vi "TETRIX Servo Move_HT_myRIO.vi"(0 "Servo Position (0 - 255)":u8(slide)=128 step=1 scale=0.0..255.0, 1 "Controller Daisy Chain Position (1 - 4)":u8=1, 3 "Enable Sync: Fast | Medium | Slow | None":string(combo)="None", 4 "Select Servo":string(combo)="Servo 1", 5 "error in (no error)":errorcluster) -> (2 "error out":errorcluster)   [LabVIEW 2014]
uses:
  <vilib>/myRIO/Instrument Drivers/Onboard IO/I2C/vis/Configure.vi
  <vilib>/myRIO/Instrument Drivers/Onboard IO/I2C/vis/Write.vi
  <vilib>/myRIO/Instrument Drivers/Onboard IO/I2C/vis/Smart Open.vi
  <vilib>/Utility/error.llb/Error Cluster From Error Code.vi
  <vilib>/myRIO/Common/Instrument Driver Framework/myRIO v1.0/I2C/vis/myRIO v1.0 Configure I2C.vi
  <vilib>/myRIO/Common/Instrument Driver Framework/myRIO v1.0/I2C/vis/myRIO v1.0 Write I2C.vi
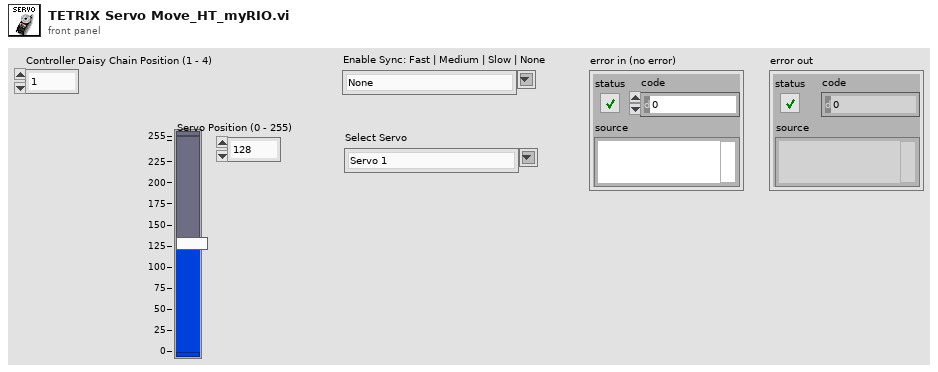
[diagram p1: front panel]
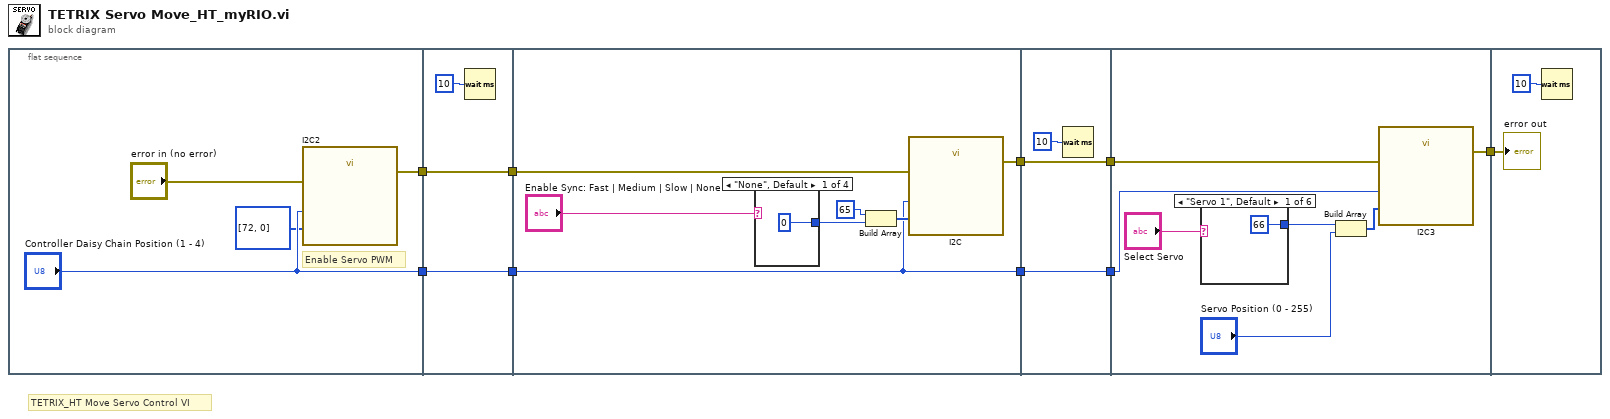
[diagram p0: block diagram]
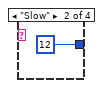
[diagram p2: hidden frame]
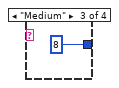
[diagram p3: hidden frame]
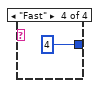
[diagram p4: hidden frame]
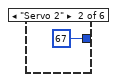
[diagram p5: hidden frame]
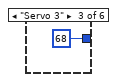
[diagram p6: hidden frame]
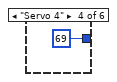
[diagram p7: hidden frame]
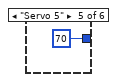
[diagram p8: hidden frame]
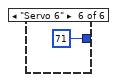
[diagram p9: hidden frame]
diagram:
  # "TETRIX_HT Move Servo Control VI"
  n1 = flat-sequence {
    tunnel: ["Controller Daisy Chain Position (1 - 4)"] -> w9
    tunnel: [w11] -> w7
    tunnel: w9 -> [w16]
    tunnel: [w16] -> w8
    tunnel: w7 -> [w15]
    tunnel: [w15] -> w6
    tunnel: [w19] -> w5
    tunnel: w8 -> [w17]
    tunnel: w6 -> [w18]
    tunnel: [w17] -> w3
    tunnel: w5 -> [w30]
    tunnel: [w30] -> w4
    tunnel: w3 -> [w29]
    tunnel: [w29] -> w2
    tunnel: w4 -> [w32]
    tunnel: w2 -> [w33]
    tunnel: [w31] -> w1
    tunnel: w1 -> [w44]
    frame #0 {
      # "Enable Servo PWM"
      n2 = call "I2C2"("Slave Address (7-bit)"="Controller Daisy Chain Position (1 - 4)", "Bytes to Write"=u8[] [72, 0], "error in (no error)"="error in (no error)") -> ("error out"=w11:errorcluster)  [unwired: 24 in]
    }
    frame #1 {
      n3 = Wait (ms)(milliseconds to wait=u32 10) -> ()  [unwired: 1 out]
    }
    frame #2 {
      n4 = case shown="\"None\", Default" "Enable Sync: Fast | Medium | Slow | None" {
        tunnel: [u8 0 u8 12 u8 8 u8 4] -> w21
        frame "None", Default {
        }
        frame "Slow" {
        }
        frame "Medium" {
        }
        frame "Fast" {
        }
      }
      n5 = Build Array(u8 65 ("element"), w21) -> (w22:u8[])
      n6 = call "I2C"("Slave Address (7-bit)"=w17, "Bytes to Write"=w22, "error in (no error)"=w18) -> ("error out"=w19:errorcluster)  [unwired: 24 in]
    }
    frame #3 {
      n7 = Wait (ms)(milliseconds to wait=u32 10) -> ()  [unwired: 1 out]
    }
    frame #4 {
      n8 = case shown="\"Servo 1\", Default" "Select Servo" {
        tunnel: [u8 66 u8 67 u8 68 u8 69 u8 70 u8 71] -> w35
        frame "Servo 1", Default {
        }
        frame "Servo 2" {
        }
        frame "Servo 3" {
        }
        frame "Servo 4" {
        }
        frame "Servo 5" {
        }
        frame "Servo 6" {
        }
      }
      n9 = Build Array(w35, "Servo Position (0 - 255)") -> (w34:u8[])
      n10 = call "I2C3"("Slave Address (7-bit)"=w33, "Bytes to Write"=w34, "error in (no error)"=w32) -> ("error out"=w31:errorcluster)  [unwired: 24 in]
    }
    frame #5 {
      n11 = Wait (ms)(milliseconds to wait=u32 10) -> ()  [unwired: 1 out]
      "error out" <- w44
    }
  }
